vi "Collect MVC.vi"(6 "Force Calibration Cluster":cluster{"Left":dbl, "Right":dbl}, 7 "Rate Hz":dbl=1000.0 format="%0.2f", 8 "error in (no error)":errorcluster, 9 "TDMS file":refnum<k34>, 10 "DAQ  Channels In":T1={"Force Transducer: Left"="Dev1/ai6", "Force Transducer: Right "="Dev1/ai8", "EMG: Left"="", "EMG: Right"="", "Potentiometer: Left"="", "Potentiometer: Right"=""}, 11 "NI Force Task in":refnum<class "NI Force Task.lvclass">) -> (0 "error out":errorcluster, 3 "NI Force Task out":refnum<class "NI Force Task.lvclass">)   [LabVIEW 2020, in "NI Force Task.lvlib" / "NI Force Task.lvclass"]
uses:
  NI Force Task.lvclass
  NI Force Task.lvclass/NI Force Task.ctl
  <vilib>/DAQmx/create/channels.llb/DAQmx Create Channel (AI-Voltage-Basic).vi
  <vilib>/DAQmx/configure/timing.llb/DAQmx Timing (Sample Clock).vi
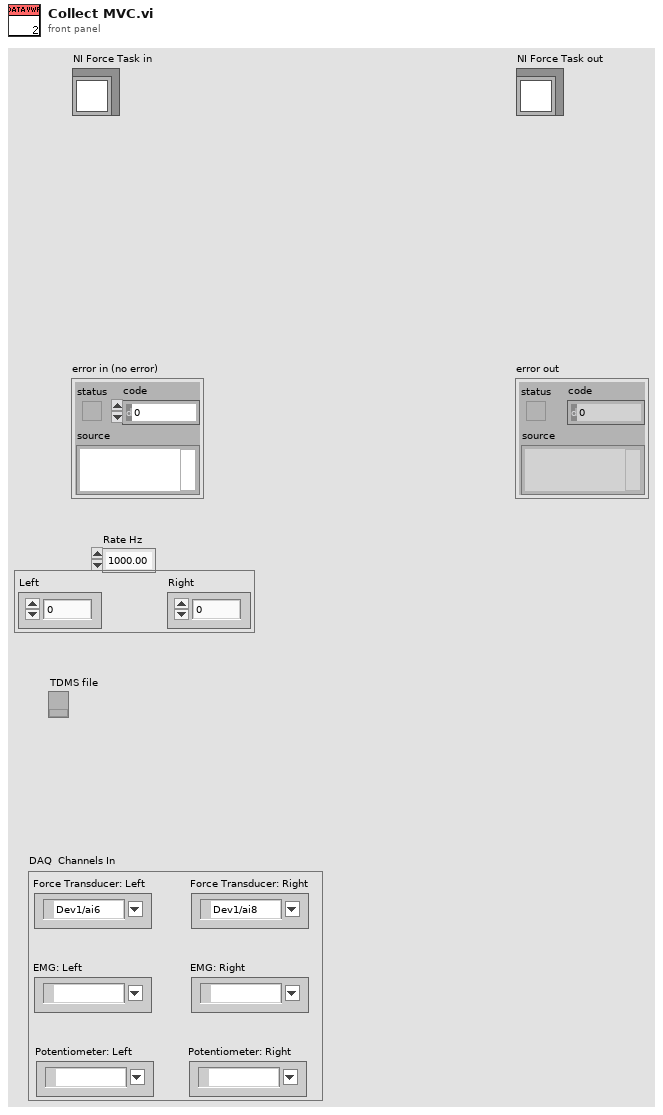
[diagram p1: front panel]
types:
  T1 = cluster{"Force Transducer: Left":tag, "Force Transducer: Right ":tag, "EMG: Left":tag, "EMG: Right":tag, "Potentiometer: Left":tag, "Potentiometer: Right":tag}
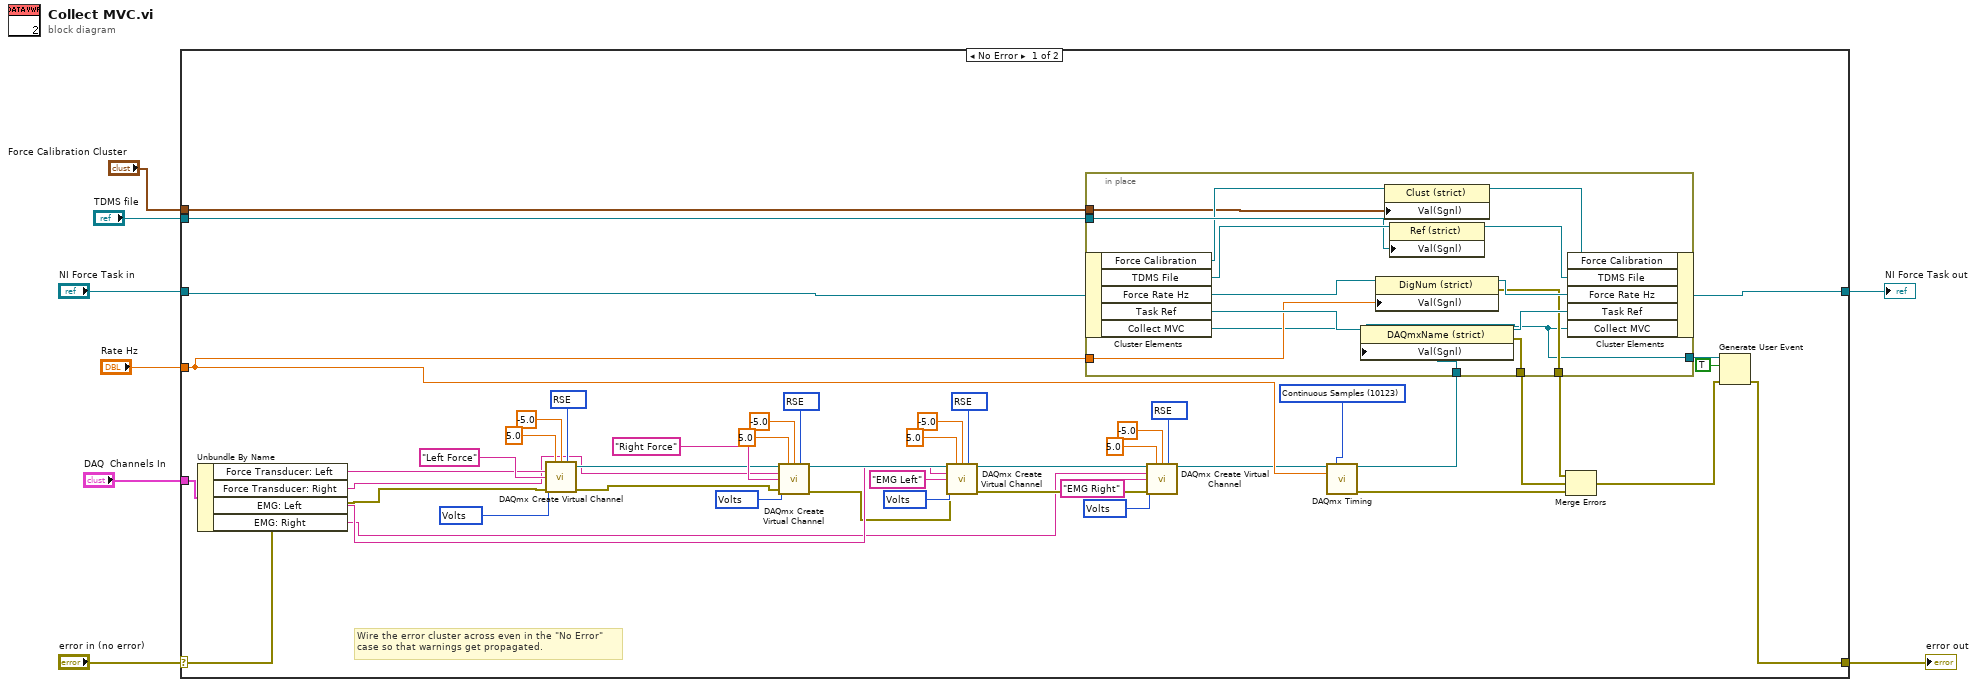
[diagram p0: block diagram]
diagram:
  n1 = case shown="No Error" "error in (no error)" {
    selector: "error in (no error)" -> [w30 w72]
    tunnel: [w29 w72] -> w7
    tunnel: [w31 w71] -> w5
    tunnel: "NI Force Task in" -> [w34 w71]
    tunnel: "Rate Hz" -> [w33 _]
    tunnel: "DAQ  Channels In" -> [w32 _]
    tunnel: "TDMS file" -> [w10 _]
    tunnel: "Force Calibration Cluster" -> [w9 _]
    frame No Error {
      w21 = 10348 items=["Volts"=10348, "From Custom Scale"=10065] ("units")
      w24 = 10083 items=["Default"=-1, "RSE"=10083, "NRSE"=10078, "Differential"=10106, "Pseudodifferential"=12529] ("input terminal configuration")
      w25 = 10348 items=["Volts"=10348, "From Custom Scale"=10065] ("units")
      w28 = 10083 items=["Default"=-1, "RSE"=10083, "NRSE"=10078, "Differential"=10106, "Pseudodifferential"=12529] ("input terminal configuration")
      w41 = 10123 items=["Finite Samples"=10178, "Continuous Samples"=10123, "Hardware Timed Single Point"=12522] ("sample mode")
      w46 = 10348 items=["Volts"=10348, "From Custom Scale"=10065] ("units")
      w50 = 10083 items=["Default"=-1, "RSE"=10083, "NRSE"=10078, "Differential"=10106, "Pseudodifferential"=12529] ("input terminal configuration")
      w51 = 10348 items=["Volts"=10348, "From Custom Scale"=10065] ("units")
      w55 = 10083 items=["Default"=-1, "RSE"=10083, "NRSE"=10078, "Differential"=10106, "Pseudodifferential"=12529] ("input terminal configuration")
      # "Wire the error cluster across even in the \"No Error\"\ncase so that warnings get propagated."
      n2 = Unbundle By Name(w32) -> ("Force Transducer: Left"=w43:tag, "Force Transducer: Right"=w42:tag, "EMG: Left"=w13:tag, "EMG: Right"=w12:tag)
      n3 = call-poly <vilib>:"DAQmx Create Virtual Channel.vi"("maximum value"=5.0, "minimum value"=-5.0, "input terminal configuration"=w55, "physical channels"=w43, "name to assign"="Left Force", "units"=w51, "error in"=w30) -> ("task out"=w45:refnum<k21>, "error out"=w44:errorcluster)  [unwired: 7 in]
      n4 = call-poly <vilib>:"DAQmx Create Virtual Channel.vi"("task in"=w45, "maximum value"=5.0, "minimum value"=-5.0, "input terminal configuration"=w50, "physical channels"=w42, "name to assign"="Right Force", "units"=w46, "error in"=w44) -> ("task out"=w16:refnum<k21>, "error out"=w11:errorcluster)  [unwired: 6 in]
      n5 = call-poly <vilib>:"DAQmx Create Virtual Channel.vi"("task in"=w16, "maximum value"=5.0, "minimum value"=-5.0, "input terminal configuration"=w28, "physical channels"=w13, "name to assign"="EMG Left", "units"=w25, "error in"=w11) -> ("task out"=w20:refnum<k21>, "error out"=w19:errorcluster)  [unwired: 6 in]
      n6 = call-poly <vilib>:"DAQmx Create Virtual Channel.vi"("task in"=w20, "maximum value"=5.0, "minimum value"=-5.0, "input terminal configuration"=w24, "physical channels"=w12, "name to assign"="EMG Right", "units"=w21, "error in"=w19) -> ("task out"=w15:refnum<k21>)  [unwired: 6 in, 1 out]
      n7 = call-poly <vilib>:"DAQmx Timing.vi"("task/channels in"=w15, "sample mode"=w41, "rate"=w33) -> ("task out"=w14:refnum<k21>, "error out"=w38:errorcluster)  [unwired: 11 in]
      n8 = in-place {
        in-place-border: w33 -> [w66]
        in-place-border: w14 -> [w65]
        in-place-border: [w64] -> w40
        in-place-border: [w63] -> w39
        in-place-border: [w62] -> w37
        in-place-border: w10 -> [w59]
        in-place-border: w9 -> [w56]
        n9 = in-place-cluster #1(w34) -> ("Force Calibration"=w58:refnum<vi>, "TDMS File"=w61:refnum<vi>, "Force Rate Hz"=w70:refnum<vi>, "Task Ref"=w68:refnum<vi>, "Collect MVC"=w62:refnum<user-event>)
        n10 = property class="DAQmxName (strict)"(reference=w68, "Val(Sgnl)"=w65) -> (reference out=w67:refnum<vi>, error out=w63:errorcluster)  [unwired: 1 in]
        n11 = property class="DigNum (strict)"(reference=w70, "Val(Sgnl)"=w66) -> (reference out=w69:refnum<vi>, error out=w64:errorcluster)  [unwired: 1 in]
        n12 = property class="Clust (strict)"(reference=w58, "Val(Sgnl)"=w56) -> (reference out=w57:refnum<vi>)  [unwired: 1 in, 1 out]
        n13 = property class="Ref (strict)"(reference=w61, "Val(Sgnl)"=w59) -> (reference out=w60:refnum<vi>)  [unwired: 1 in, 1 out]
        n14 = in-place-cluster #1("Force Calibration"=w57, "TDMS File"=w60, "Force Rate Hz"=w69, "Task Ref"=w67, "Collect MVC"=w62) -> (w31:refnum<class "NI Force Task.lvclass">)
      }
      n15 = Merge Errors(w40, w39, w38) -> (w35:errorcluster)
      n16 = Generate User Event(user event=w37, event data cluster=TRUE ("event data"), error in=w35) -> (error out=w29:errorcluster)  [unwired: 1 in, 1 out]
    }
    frame Error {
    }
  }
  "error out" <- w7
  "NI Force Task out" <- w5
